vi "mClampMPI.vi"() -> ()   [LabVIEW 2011]
uses:
  <vilib>/DAQmx/write.llb/DAQmx Write (Analog 1D Wfm NChan NSamp).vi
  <vilib>/DAQmx/read.llb/DAQmx Read (Analog 1D Wfm NChan NSamp).vi
  <vilib>/DAQmx/create/channels.llb/DAQmx Create Channel (AO-Voltage-Basic).vi
  <vilib>/DAQmx/configure/timing.llb/DAQmx Timing (Sample Clock).vi
  <vilib>/DAQmx/create/channels.llb/DAQmx Create Channel (AI-Voltage-Basic).vi
  <vilib>/DAQmx/miscellaneous.llb/DAQmx Fill In Error Info.vi
  <vilib>/ptbypt/NI_PtbyPt.lvlib
panel:
  in  "Amplitude (nA)":dbl=2.0
  out "Waveform Chart 2":dynamicdata(graph)
  in  "Voltage Clamp":bool=TRUE
  out "resistance (MOhm)":dbl
  out "Off":bool
  out "On":bool
  in  "Amplitude (mV)":dbl=10.0
  in  "R test":bool
  in  "Off Time (msec)":u32=1000
  in  "On Time (msec)":u32=100
  in  "stop":bool
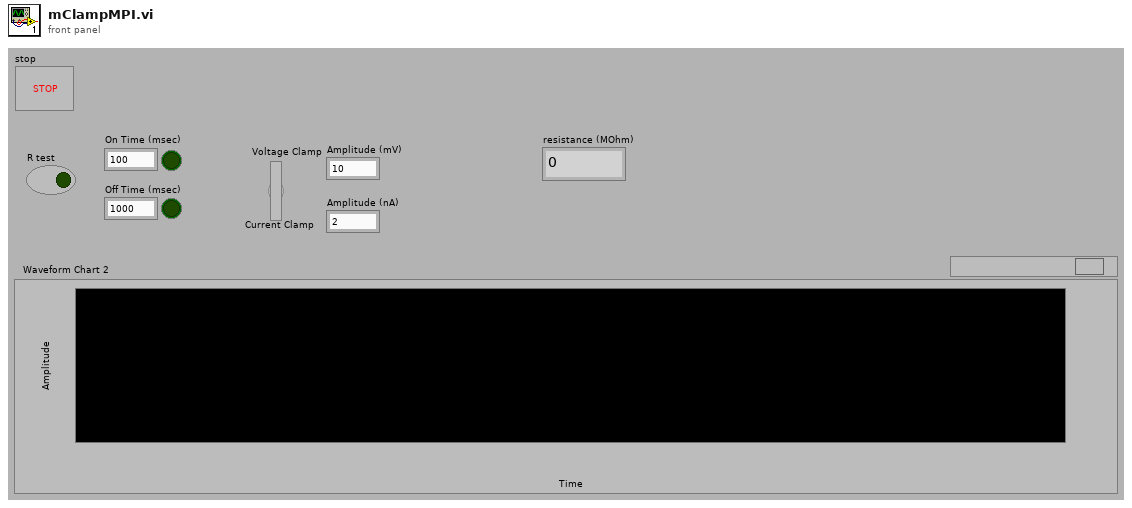
[diagram p1: front panel]
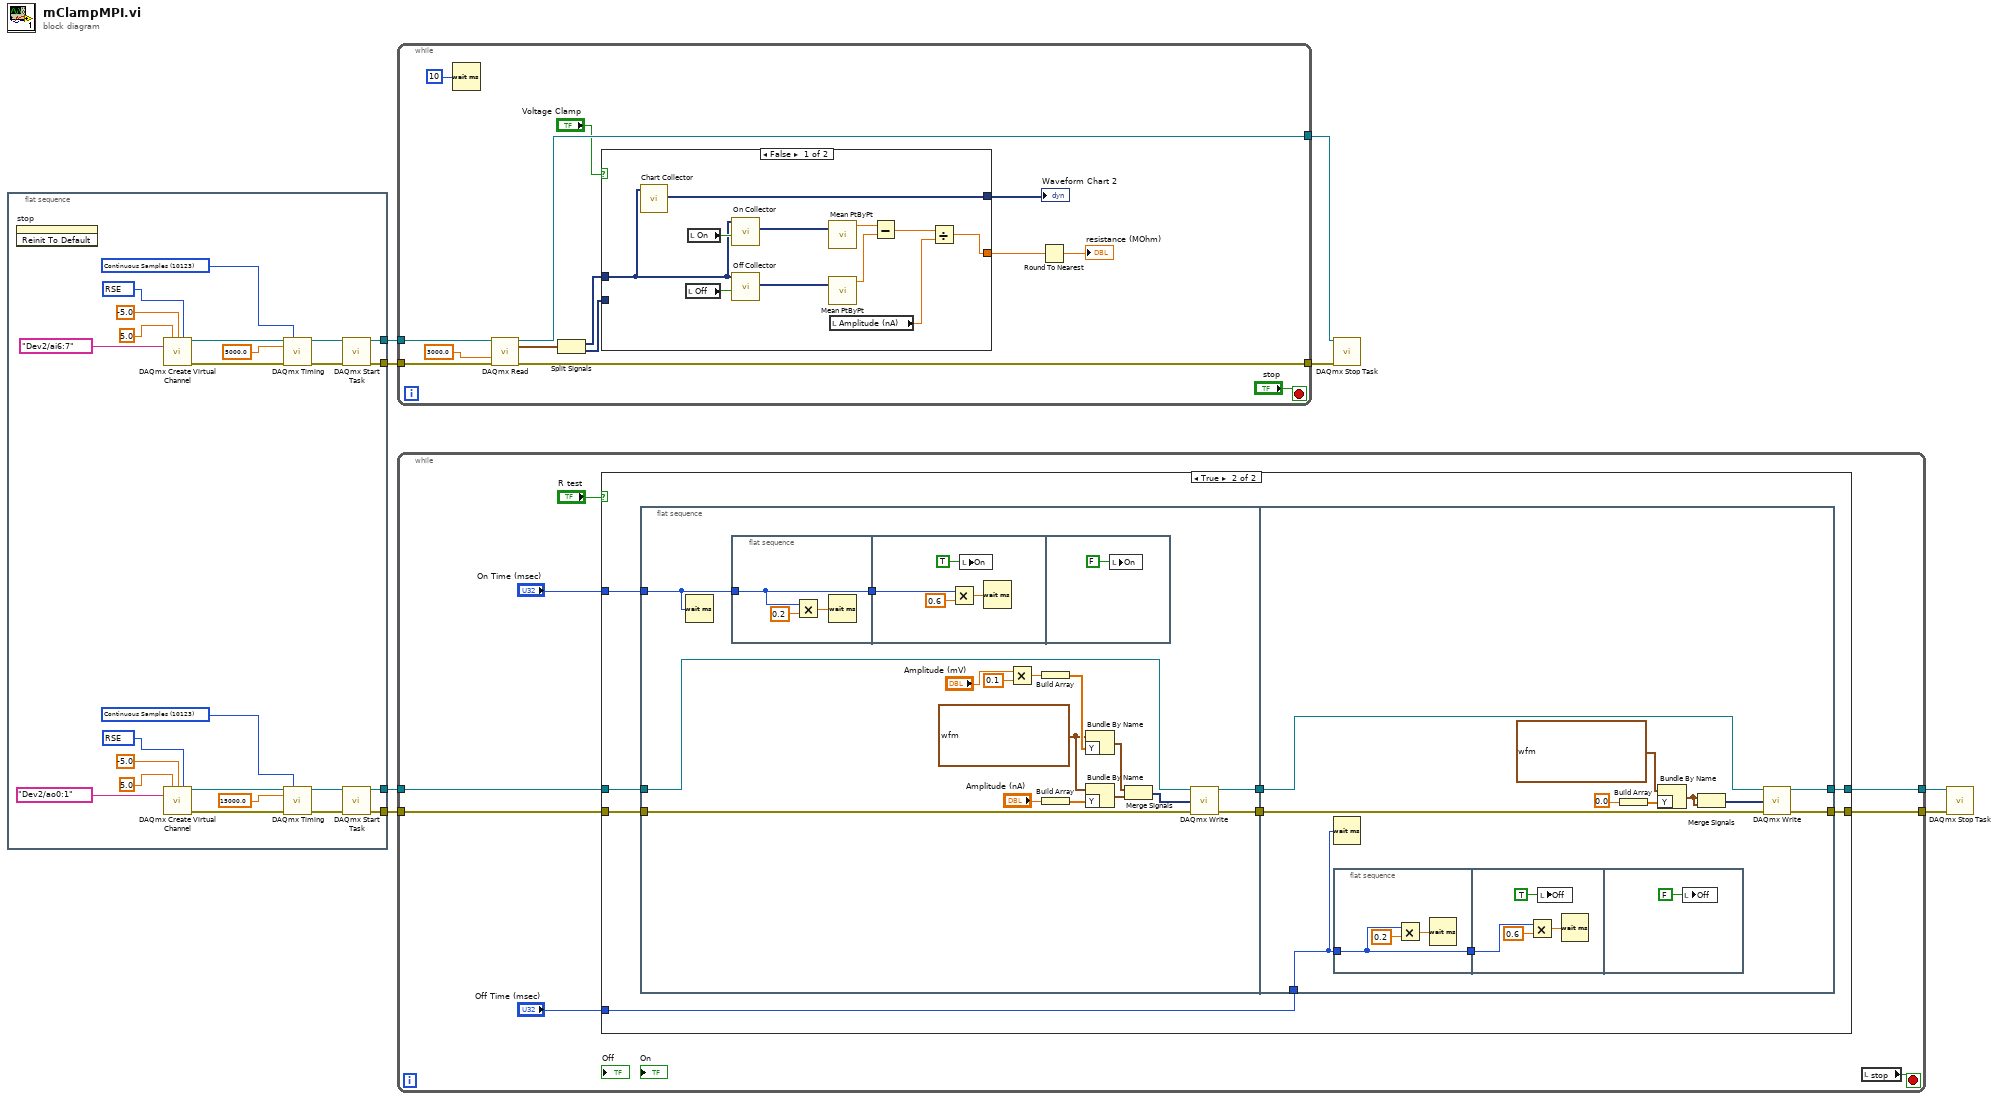
[diagram p0: block diagram]
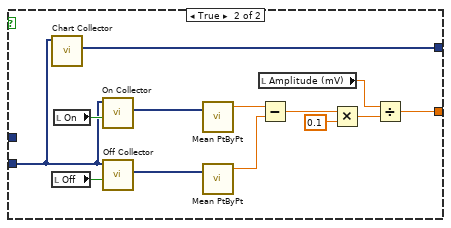
[diagram p3: hidden frame]
diagram:
  n1 = flat-sequence {
    tunnel: [w24] -> w8
    tunnel: [w23] -> w7
    tunnel: [w10] -> w4
    tunnel: [w9] -> w3
    frame #0 {
      w20 = 10083 items=["default"=-1, "RSE"=10083, "NRSE"=10078, "Differential"=10106, "Pseudodifferential"=12529] ("input terminal configuration")
      w16 = 10123 items=["Finite Samples"=10178, "Continuous Samples"=10123, "Hardware Timed Single Point"=12522] ("sample mode")
      w21 = 10083 items=["default"=-1, "RSE"=10083, "NRSE"=10078, "Differential"=10106, "Pseudodifferential"=12529] ("input terminal configuration")
      w28 = 10123 items=["Finite Samples"=10178, "Continuous Samples"=10123, "Hardware Timed Single Point"=12522] ("sample mode")
      n2 = invoke on="stop" class="Bool (strict)" method="Reinit To Default"() -> ()  [unwired: 3 in, 3 out]
      n3 = call-poly <vilib>:"DAQmx Create Virtual Channel.vi"("maximum value"=5.0, "minimum value"=-5.0, "input terminal configuration"=w21, "physical channels"=tag "Dev2/ai6:7") -> ("task out"=w30:refnum<k21>, "error out"=w29:errorcluster)  [unwired: 10 in]
      n4 = call-poly <vilib>:"DAQmx Create Virtual Channel.vi"("maximum value"=5.0, "minimum value"=-5.0, "output terminal configuration"=w20, "physical channels"=tag "Dev2/ao0:1" ("physical channels 2")) -> ("task out"=w14:refnum<k21>, "error out"=w15:errorcluster)  [unwired: 10 in]
      n5 = call-poly <vilib>:"DAQmx Timing.vi"("task/channels in"=w30, "sample mode"=w28, "rate"=5000.0, "error in"=w29) -> ("task out"=w32:refnum<k21>, "error out"=w31:errorcluster)  [unwired: 10 in]
      n6 = call-poly <vilib>:"DAQmx Timing.vi"("task/channels in"=w14, "sample mode"=w16, "rate"=15000.0, "error in"=w15) -> ("task out"=w12:refnum<k21>, "error out"=w13:errorcluster)  [unwired: 10 in]
      n7 = call <vilib>:"DAQmx Start Task.vi"("task/channels in"=w32, "error in"=w31) -> ("task out"=w24:refnum<k21>, "error out"=w23:errorcluster)  [unwired: 12 in]
      n8 = call <vilib>:"DAQmx Start Task.vi"("task/channels in"=w12, "error in"=w13) -> ("task out"=w10:refnum<k21>, "error out"=w9:errorcluster)  [unwired: 12 in]
    }
  }
  n9 = while {
    tunnel: w8 -> [w42]
    tunnel: w7 -> [w41]
    tunnel: [w40] -> w2
    tunnel: [w39] -> w1
    stop <- "stop" stop-if-true
    n10 = Wait (ms)(milliseconds to wait=u32 10) -> ()  [unwired: 1 out]
    n11 = call-poly <vilib>:"DAQmx Read.vi"("task/channels in"=w42, "timeout"=3000.0, "error in"=w41) -> ("task out"=w40:refnum<k21>, "data"=w37:waveform(dbl)[], "error out"=w39:errorcluster)  [unwired: 10 in]
    n12 = Split Signals(w37) -> (w36:dynamicdata, w35:dynamicdata)  [unwired: 2 in]
    n13 = case shown="False" "Voltage Clamp" {
      tunnel: [w51 w60] -> w44
      tunnel: [w50 w59] -> w34
      tunnel: w36 -> [w49 _]
      tunnel: w35 -> [_ w58]
      frame False {
        n14 = call "Chart Collector"("Signals"=w49) -> ("Collected Signals"=w51:dynamicdata)  [unwired: 9 in, 1 out]
        n15 = local read "Off"() -> (w56:bool)
        n16 = local read "On"() -> (w57:bool)
        n17 = call "On Collector"("Enable"=w57, "Signals"=w49) -> ("Collected Signals"=w55:dynamicdata)  [unwired: 8 in, 1 out]
        n18 = call "Off Collector"("Enable"=w56, "Signals"=w49) -> ("Collected Signals"=w54:dynamicdata)  [unwired: 8 in, 1 out]
        n19 = call <vilib>:"Mean PtByPt.vi"("x"=w55) -> ("mean"=w53:dbl)  [unwired: 3 in, 1 out]
        n20 = call <vilib>:"Mean PtByPt.vi"("x"=w54) -> ("mean"=w52:dbl)  [unwired: 3 in, 1 out]
        n21 = local read "Amplitude (nA)"() -> (w48:dbl)
        n22 = Subtract(x=w53, y=w52) -> (x-y=w47:dbl)
        n23 = Divide(x=w47, y=w48) -> (x/y=w50:dbl)
      }
      frame True {
        n24 = call "Chart Collector"("Signals"=w58) -> ("Collected Signals"=w60:dynamicdata)  [unwired: 9 in, 1 out]
        n25 = local read "Off"() -> (w69:bool)
        n26 = local read "On"() -> (w70:bool)
        n27 = call "On Collector"("Enable"=w70, "Signals"=w58) -> ("Collected Signals"=w68:dynamicdata)  [unwired: 8 in, 1 out]
        n28 = call "Off Collector"("Enable"=w69, "Signals"=w58) -> ("Collected Signals"=w67:dynamicdata)  [unwired: 8 in, 1 out]
        n29 = call <vilib>:"Mean PtByPt.vi"("x"=w68) -> ("mean"=w66:dbl)  [unwired: 3 in, 1 out]
        n30 = call <vilib>:"Mean PtByPt.vi"("x"=w67) -> ("mean"=w65:dbl)  [unwired: 3 in, 1 out]
        n31 = local read "Amplitude (mV)"() -> (w61:dbl)
        n32 = Subtract(x=w66, y=w65) -> (x-y=w64:dbl)
        n33 = Multiply(x=w64, y=0.1) -> (x*y=w62:dbl)
        n34 = Divide(x=w61, y=w62) -> (x/y=w59:dbl)
      }
    }
    "Waveform Chart 2" <- w44
    n35 = Round To Nearest(number=w34) -> (nearest integer value=→"resistance (MOhm)":dbl)
  }
  n36 = while {
    tunnel: [w77] -> w6
    tunnel: [w71] -> w5
    tunnel: w4 -> [w73]
    tunnel: w3 -> [w72]
    stop <- w78 stop-if-true
    n37 = case shown="True" "R test" {
      tunnel: [w80 w86] -> w77
      tunnel: "On Time (msec)" -> [_ w85]
      tunnel: "Off Time (msec)" -> [_ w84]
      tunnel: w73 -> [w80 w83]
      tunnel: w72 -> [w79 w82]
      tunnel: [w79 w81] -> w71
      frame False {
      }
      frame True {
        n38 = flat-sequence {
          tunnel: [w104] -> w88
          tunnel: [w103] -> w87
          tunnel: w85 -> [w97]
          tunnel: w83 -> [w96]
          tunnel: w82 -> [w95]
          tunnel: w88 -> [w123]
          tunnel: w87 -> [w122]
          tunnel: [w121] -> w86
          tunnel: [w120] -> w81
          tunnel: w84 -> [w116]
          frame #0 {
            w93 = waveform(dbl) {"t0"=timestamp(0 s since 1904-01-01), "dt"=1.0, "Y"=[]} ("Waveform")
            n39 = Wait (ms)(milliseconds to wait=w97) -> ()  [unwired: 1 out]
            n40 = flat-sequence {
              tunnel: w97 -> [w105]
              tunnel: [w105] -> w101
              tunnel: w101 -> [w108]
              frame #0 {
                n41 = Multiply(x=w105, y=0.2) -> (x*y=w107:dbl)
                n42 = Wait (ms)(milliseconds to wait=w107) -> ()  [unwired: 1 out]
              }
              frame #1 {
                n43 = Multiply(x=w108, y=0.6) -> (x*y=w109:dbl)
                n44 = local write "On"(TRUE) -> ()
                n45 = Wait (ms)(milliseconds to wait=w109) -> ()  [unwired: 1 out]
              }
              frame #2 {
                n46 = local write "On"(FALSE ("Detect")) -> ()
              }
            }
            n47 = Multiply(x="Amplitude (mV)", y=0.1) -> (x*y=w100:dbl)
            n48 = Build Array(w100) -> (w102:dbl[])
            n49 = Build Array("Amplitude (nA)") -> (w94:dbl[])
            n50 = Bundle By Name(cluster=w93, "Y"=w102) -> (w91:waveform(dbl))
            n51 = Bundle By Name(cluster=w93, "Y"=w94) -> (w92:waveform(dbl))
            n52 = Merge Signals(w91, w92) -> (w90:dynamicdata)
            n53 = call-poly <vilib>:"DAQmx Write.vi"("task/channels in"=w96, "data"=w90, "error in"=w95) -> ("task out"=w104:refnum<k21>, "error out"=w103:errorcluster)  [unwired: 10 in, 1 out]
          }
          frame #1 {
            n54 = Wait (ms)(milliseconds to wait=w116) -> ()  [unwired: 1 out]
            n55 = flat-sequence {
              tunnel: w116 -> [w124]
              tunnel: [w124] -> w117
              tunnel: w117 -> [w127]
              frame #0 {
                n56 = Multiply(x=w124, y=0.2) -> (x*y=w126:dbl)
                n57 = Wait (ms)(milliseconds to wait=w126) -> ()  [unwired: 1 out]
              }
              frame #1 {
                n58 = Multiply(x=w127, y=0.6) -> (x*y=w128:dbl)
                n59 = local write "Off"(TRUE) -> ()
                n60 = Wait (ms)(milliseconds to wait=w128) -> ()  [unwired: 1 out]
              }
              frame #2 {
                n61 = local write "Off"(FALSE ("Detect")) -> ()
              }
            }
            n62 = Build Array(0.0) -> (w118:dbl[])
            n63 = Bundle By Name(cluster=waveform(dbl) {"t0"=timestamp(0 s since 1904-01-01), "dt"=1.0, "Y"=[]} ("Waveform"), "Y"=w118) -> (w114:waveform(dbl))
            n64 = Merge Signals(w114, w114) -> (w113:dynamicdata)
            n65 = call-poly <vilib>:"DAQmx Write.vi"("task/channels in"=w123, "data"=w113, "error in"=w122) -> ("task out"=w121:refnum<k21>, "error out"=w120:errorcluster)  [unwired: 10 in, 1 out]
          }
        }
      }
    }
    n66 = local read "stop"() -> (w78:bool)
  }
  n67 = call <vilib>:"DAQmx Stop Task.vi"("task/channels in"=w2, "error in"=w1) -> ()  [unwired: 12 in, 2 out]
  n68 = call <vilib>:"DAQmx Stop Task.vi"("task/channels in"=w6, "error in"=w5) -> ()  [unwired: 12 in, 2 out]
